vi "GPStest.vi"() -> ()   [LabVIEW 2019]
uses:
  <vilib>/LabVIEW Open Source Project/Data Manipulation/Scalar/FinalStringFormatting.vi
  <vilib>/Instr/_visa.llb/VISA Configure Serial Port (Instr).vi
  <vilib>/LabVIEW Open Source Project/Data Manipulation/Scalar/Get Decimal Separator.vi
  <vilib>/Utility/file.llb/Write Delimited Spreadsheet (string).vi
  <vilib>/LabVIEW Open Source Project/Data Manipulation/Scalar/OpenScalar.lvlib
panel:
  out "GPGSV":string
  out "number of message":string
  out "msg1":string
  out "Satelite in view":string
  in  "Satelite_id/elevation/azimuth/SNR 17":enum32{"Msg 1", "Msg 2", "Msg 3", "Msg 4"}(tab)
  out "Satelite_id/elevation/azimuth/SNR":string[](array[string])
  out "Satelite_id/elevation/azimuth/SNR 2":string[](array[string])
  out "Satelite_id/elevation/azimuth/SNR 3":string[](array[string])
  out "Satelite_id/elevation/azimuth/SNR 4":string[](array[string])
  out "Signal ID / Check sum":string[](array[string])
  out "Signal ID / Check sum 2":string[](array[string])
  out "Satelite_id/elevation/azimuth/SNR 8":string[](array[string])
  out "Satelite_id/elevation/azimuth/SNR 7":string[](array[string])
  out "Satelite_id/elevation/azimuth/SNR 6":string[](array[string])
  out "Satelite_id/elevation/azimuth/SNR 5":string[](array[string])
  out "Signal ID / Check sum 3":string[](array[string])
  out "Satelite_id/elevation/azimuth/SNR 12":string[](array[string])
  out "Satelite_id/elevation/azimuth/SNR 11":string[](array[string])
  out "Satelite_id/elevation/azimuth/SNR 10":string[](array[string])
  out "Satelite_id/elevation/azimuth/SNR 9":string[](array[string])
  out "Signal ID / Check sum 4":string[](array[string])
  out "Satelite_id/elevation/azimuth/SNR 16":string[](array[string])
  out "Satelite_id/elevation/azimuth/SNR 15":string[](array[string])
  out "Satelite_id/elevation/azimuth/SNR 14":string[](array[string])
  out "Satelite_id/elevation/azimuth/SNR 13":string[](array[string])
  out "GSA":string
  out "Operation Mode":string
  out "Navigation mode":string
  out "satelite used channel 1":string
  out "satelite used channel 2":string
  out "satelite used channel 3":string
  out "satelite used channel 4":string
  out "satelite used channel 5":string
  out "satelite used channel 6":string
  out "satelite used channel 7":string
  out "satelite used channel 8":string
  out "satelite used channel 9":string
  out "satelite used channel 10":string
  out "satelite used channel 11":string
  out "satelite used channel 12":string
  out "pdop":string
  out "hdop 2":string
  out "vdop":string
  out "System ID":string
  out "Checksum 3":string
  out "GGA 3":string
  out "UTC time":string
  out "Lat 3":string
  out "NS 2":string
  out "Long 2":string
  out "EW 2":string
  out "Pos_indicator":string
  out "Number of Satelite_used":string
  out "hdop":string
  out "msl_altitude":string
  out "altitude_units":string
  out "geoidal_Seperation":string
  out "Separation unit":string
  out "age of Diff corr":string
  out "diffStating":string
  out "Checksum 2":string
  out "VTG":string
  out "Course over Ground":string
  out "Reference":string
  out "Course over Ground (Magnetic)":string
  out "Reference2":string
  out "Speedover Ground (knots)":string
  out "Units1":string
  out "Speed over ground kph":string
  out "Units 2":string
  out "Position Mode 2":string
  out "Check sum 2":string
  out "Lat 2":string
  out "NS":string
  out "GLL":string
  out "Long 3":string
  out "EW":string
  out "Time":string
  out "Status 2":string
  out "Positioning mod":string
  out "Check sum":string
  out "Carriage return 2":string
  out "GBGSV 4":string
  out "number of message 4":string
  out "msg1 4":string
  out "Satelite in view 4":string
  in  "Satelite_id/elevation/azimuth/SNR 68":enum32{"Msg 1", "Msg 2", "Msg 3", "Msg 4"}(tab)
  out "Satelite_id/elevation/azimuth/SNR 55":string[](array[string])
  out "Satelite_id/elevation/azimuth/SNR 54":string[](array[string])
  out "Satelite_id/elevation/azimuth/SNR 53":string[](array[string])
  out "Satelite_id/elevation/azimuth/SNR 52":string[](array[string])
  out "Signal ID / Check sum 13":string[](array[string])
  out "Signal ID / Check sum 14":string[](array[string])
  out "Satelite_id/elevation/azimuth/SNR 59":string[](array[string])
  out "Satelite_id/elevation/azimuth/SNR 56":string[](array[string])
  out "Satelite_id/elevation/azimuth/SNR 57":string[](array[string])
  out "Satelite_id/elevation/azimuth/SNR 58":string[](array[string])
  out "Signal ID / Check sum 15":string[](array[string])
  out "Satelite_id/elevation/azimuth/SNR 63":string[](array[string])
  out "Satelite_id/elevation/azimuth/SNR 60":string[](array[string])
  out "Satelite_id/elevation/azimuth/SNR 61":string[](array[string])
  out "Satelite_id/elevation/azimuth/SNR 62":string[](array[string])
  out "Signal ID / Check sum 16":string[](array[string])
  out "Satelite_id/elevation/azimuth/SNR 67":string[](array[string])
  out "Satelite_id/elevation/azimuth/SNR 64":string[](array[string])
  out "Satelite_id/elevation/azimuth/SNR 65":string[](array[string])
  out "Satelite_id/elevation/azimuth/SNR 66":string[](array[string])
  out "GAGSV 3":string
  out "number of message 3":string
  out "msg1 3":string
  out "Satelite in view 3":string
  in  "Satelite_id/elevation/azimuth/SNR 51":enum32{"Msg 1", "Msg 2", "Msg 3", "Msg 4"}(tab)
  out "Satelite_id/elevation/azimuth/SNR 38":string[](array[string])
  out "Satelite_id/elevation/azimuth/SNR 37":string[](array[string])
  out "Satelite_id/elevation/azimuth/SNR 36":string[](array[string])
  out "Satelite_id/elevation/azimuth/SNR 35":string[](array[string])
  out "Signal ID / Check sum 9":string[](array[string])
  out "Signal ID / Check sum 10":string[](array[string])
  out "Satelite_id/elevation/azimuth/SNR 42":string[](array[string])
  out "Satelite_id/elevation/azimuth/SNR 39":string[](array[string])
  out "Satelite_id/elevation/azimuth/SNR 40":string[](array[string])
  out "Satelite_id/elevation/azimuth/SNR 41":string[](array[string])
  out "Signal ID / Check sum 11":string[](array[string])
  out "Satelite_id/elevation/azimuth/SNR 46":string[](array[string])
  out "Satelite_id/elevation/azimuth/SNR 43":string[](array[string])
  out "Satelite_id/elevation/azimuth/SNR 44":string[](array[string])
  out "Satelite_id/elevation/azimuth/SNR 45":string[](array[string])
  out "Signal ID / Check sum 12":string[](array[string])
  out "Satelite_id/elevation/azimuth/SNR 50":string[](array[string])
  out "Satelite_id/elevation/azimuth/SNR 47":string[](array[string])
  out "Satelite_id/elevation/azimuth/SNR 48":string[](array[string])
  out "Satelite_id/elevation/azimuth/SNR 49":string[](array[string])
  out "GLGSV 2":string
  out "number of message 2":string
  out "msg1 2":string
  out "Satelite in view 2":string
  in  "Satelite_id/elevation/azimuth/SNR 34":enum32{"Msg 1", "Msg 2", "Msg 3", "Msg 4"}(tab)
  out "Satelite_id/elevation/azimuth/SNR 21":string[](array[string])
  out "Satelite_id/elevation/azimuth/SNR 20":string[](array[string])
  out "Satelite_id/elevation/azimuth/SNR 19":string[](array[string])
  out "Satelite_id/elevation/azimuth/SNR 18":string[](array[string])
  out "Signal ID / Check sum 5":string[](array[string])
  out "Signal ID / Check sum 6":string[](array[string])
  out "Satelite_id/elevation/azimuth/SNR 25":string[](array[string])
  out "Satelite_id/elevation/azimuth/SNR 22":string[](array[string])
  out "Satelite_id/elevation/azimuth/SNR 23":string[](array[string])
  out "Satelite_id/elevation/azimuth/SNR 24":string[](array[string])
  out "Signal ID / Check sum 7":string[](array[string])
  out "Satelite_id/elevation/azimuth/SNR 29":string[](array[string])
  out "Satelite_id/elevation/azimuth/SNR 26":string[](array[string])
  out "Satelite_id/elevation/azimuth/SNR 27":string[](array[string])
  out "Satelite_id/elevation/azimuth/SNR 28":string[](array[string])
  out "Signal ID / Check sum 8":string[](array[string])
  out "Satelite_id/elevation/azimuth/SNR 33":string[](array[string])
  out "Satelite_id/elevation/azimuth/SNR 30":string[](array[string])
  out "Satelite_id/elevation/azimuth/SNR 31":string[](array[string])
  out "Satelite_id/elevation/azimuth/SNR 32":string[](array[string])
  out "UTC Time":string
  out "Status":string
  out "Lat":string
  out "N/S":string
  out "Long":string
  out "E/W":string
  out "Speed over ground[knot]":string
  out "Course over Ground [Degrees]":string
  out "date[ddmmyy]":string
  out "Mode":string
  out "xxRMC":string
  out "NavStatus":string
  out "Checksum":string
  out "Carriage return":string
  in  "stop":bool
  in  "error in (no error) 2":errorcluster
  out "read buffer":string
  out "Array":string[](array[string])
  out "VISA Refnum":refnum<visa-resource-name>
  out "error out":errorcluster
  out "Raw output from GPS":string
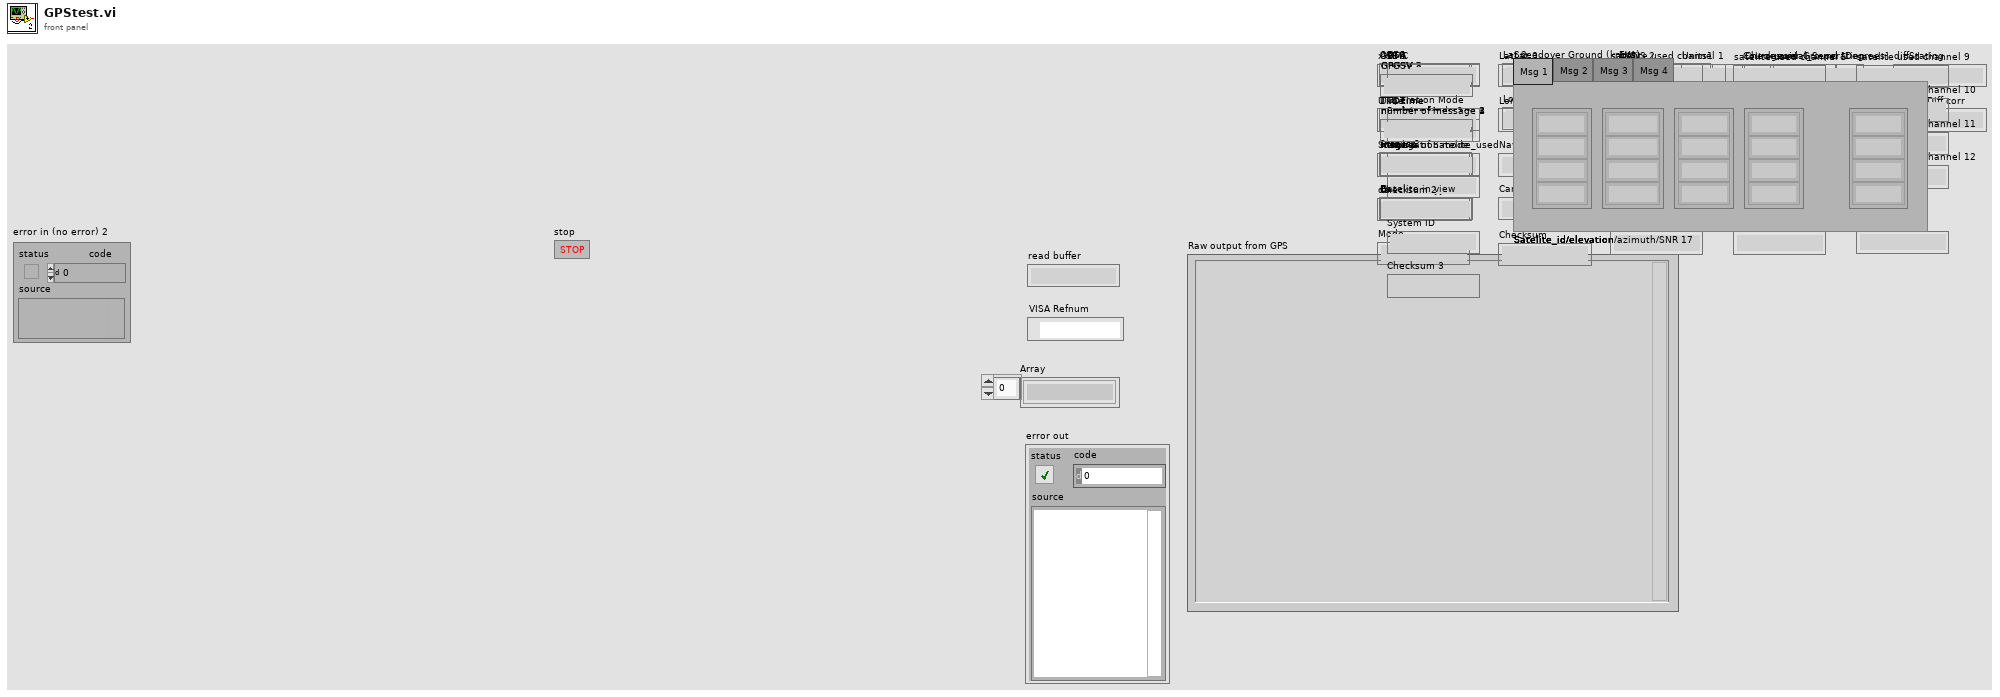
[diagram p1: front panel]
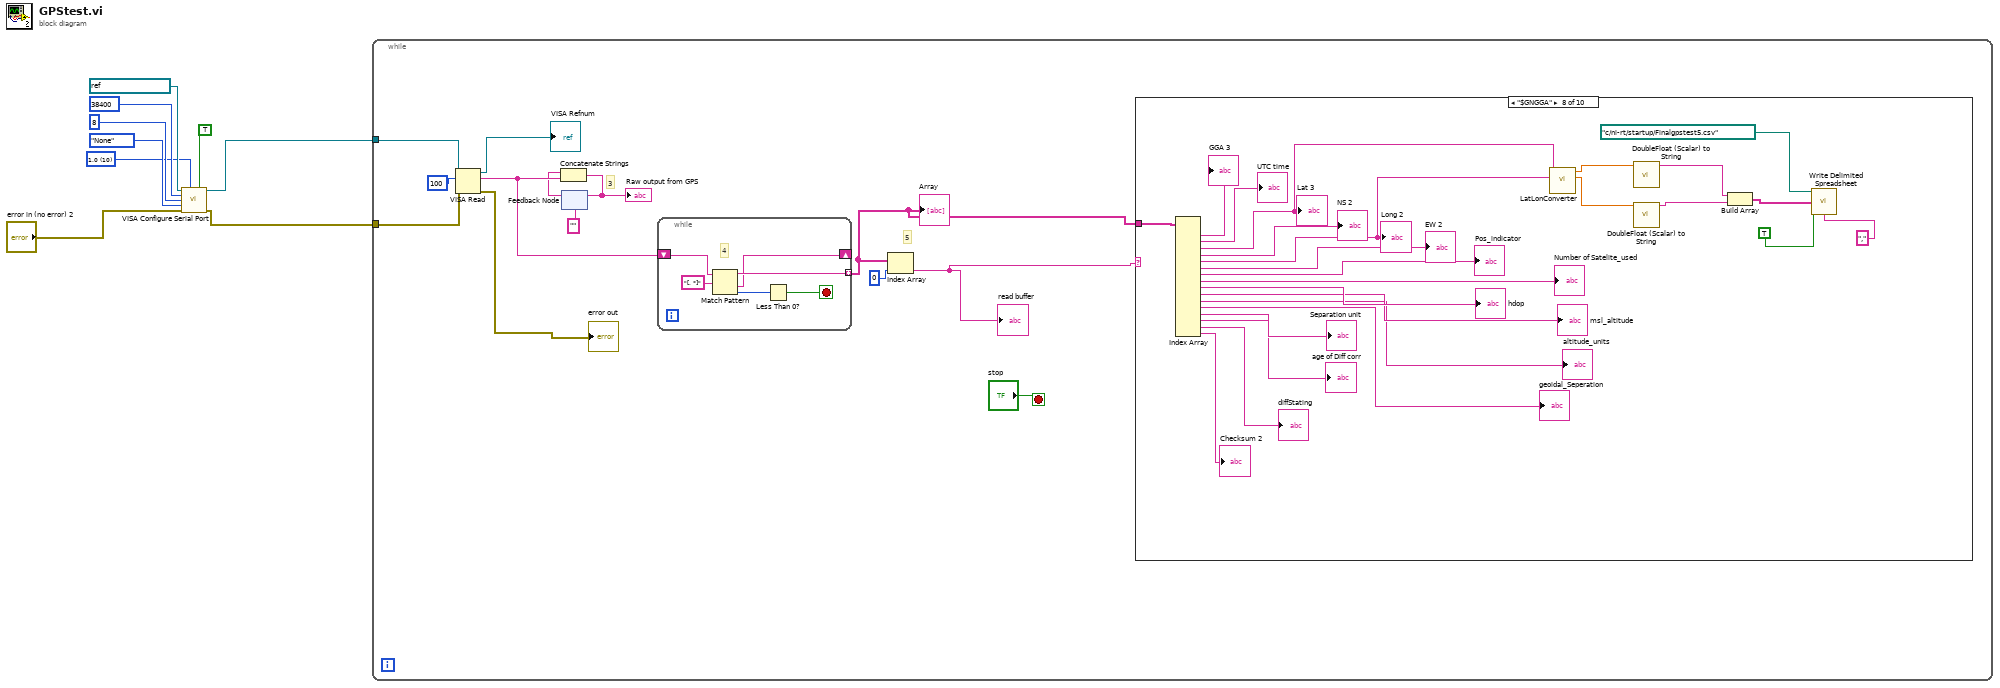
[diagram p0: block diagram]
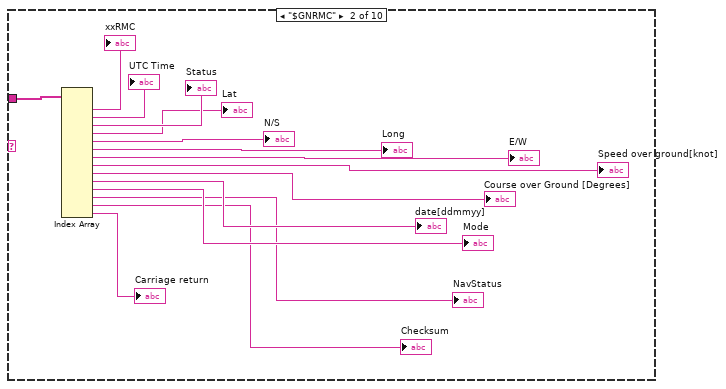
[diagram p3: hidden frame]
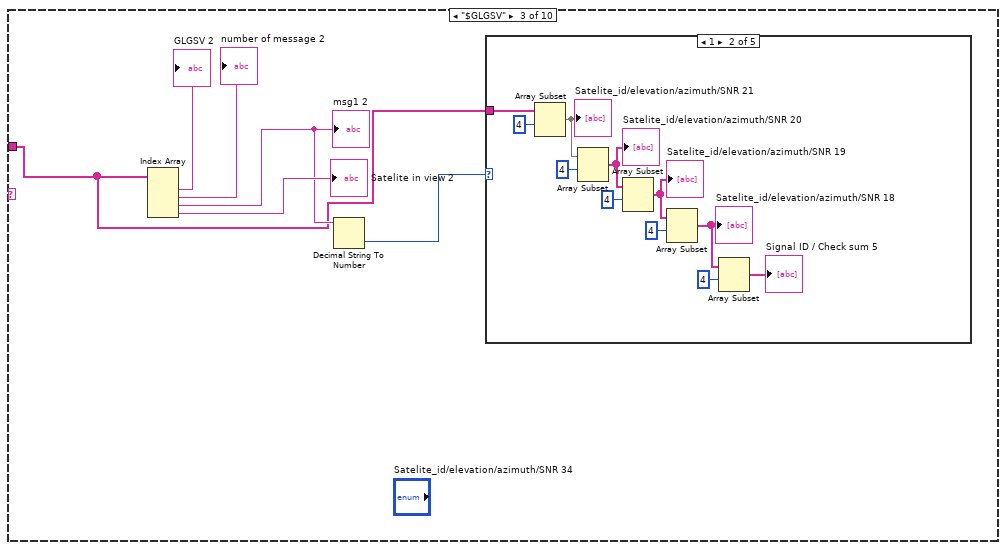
[diagram p4: hidden frame]
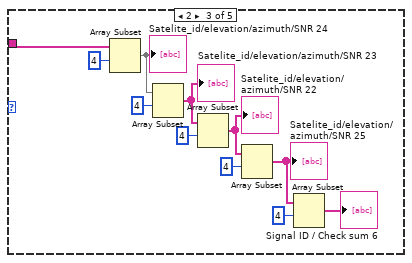
[diagram p6: hidden frame]
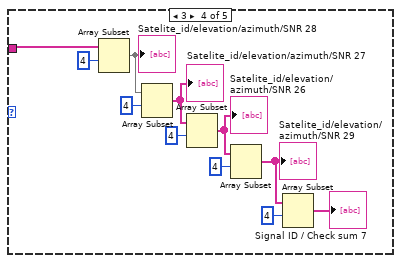
[diagram p7: hidden frame]
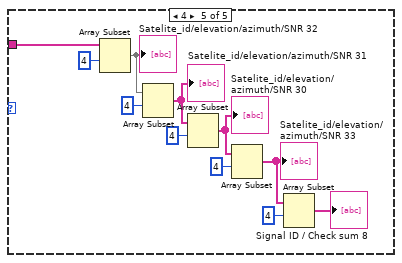
[diagram p8: hidden frame]
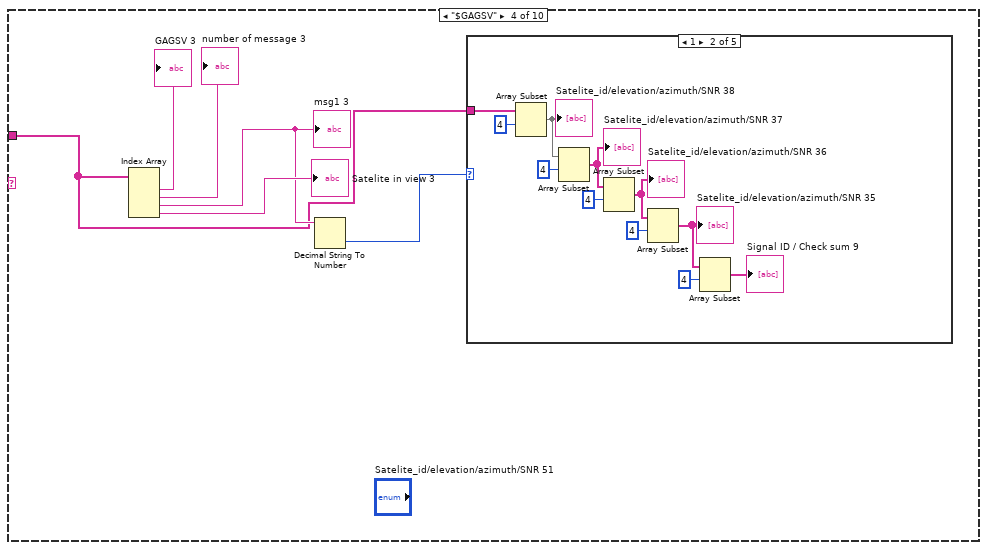
[diagram p9: hidden frame]
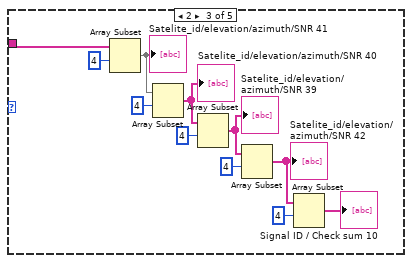
[diagram p11: hidden frame]
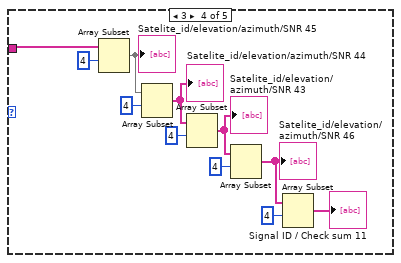
[diagram p12: hidden frame]
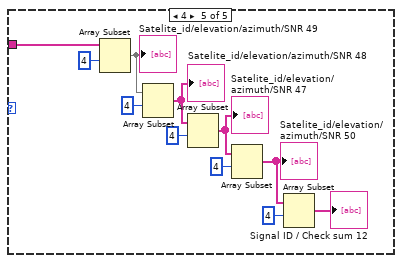
[diagram p13: hidden frame]
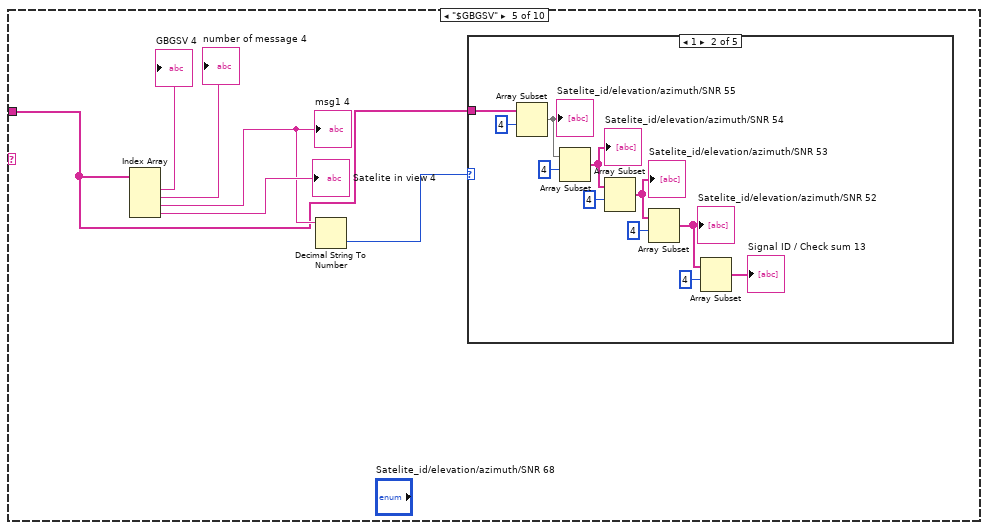
[diagram p14: hidden frame]
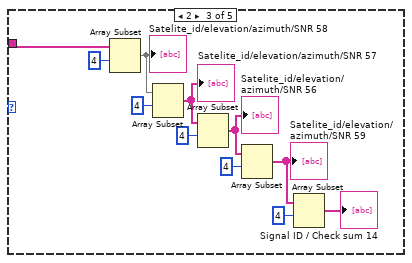
[diagram p16: hidden frame]
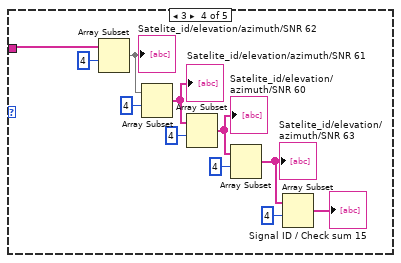
[diagram p17: hidden frame]
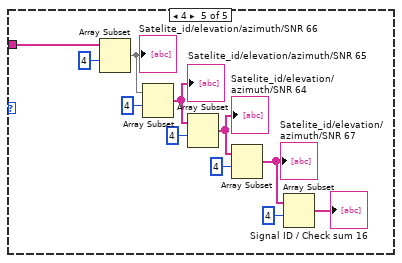
[diagram p18: hidden frame]
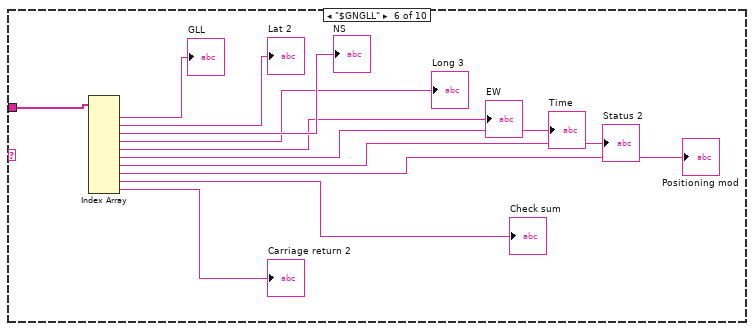
[diagram p19: hidden frame]
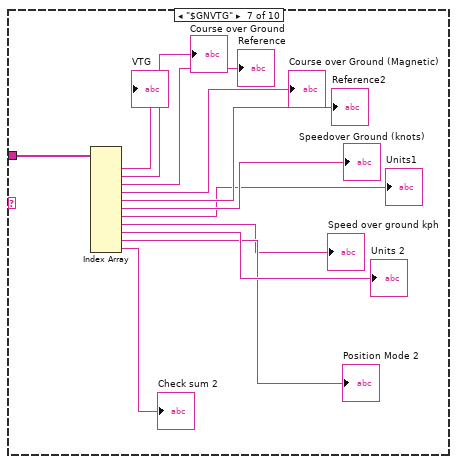
[diagram p20: hidden frame]
diagram:
  w4 = u16 10 items=["1.0"=10, "1.5"=15, "2.0"=20] ("stop bits (10: 1 bit)")
  n1 = call-poly "VISA Configure Serial Port"("VISA resource name"=refnum<visa-resource-name> "ASRL1::INSTR", "Enable Termination\nChar (T)"=TRUE ("Enable Termination\nChar (T)"), "baud rate (9600)"=u32 38400, "data bits (8)"=u16 8, "parity (0:none)"=enum16{"None", "Odd", "Even", "Mark", "Space"}."None", "error in (no error)"="error in (no error) 2", "stop bits (10: 1 bit)"=w4) -> ("VISA resource name out"=w3:refnum<visa-resource-name>, "error out"=w1:errorcluster)  [unwired: 7 in]
  n2 = while {
    tunnel: w3 -> [w15]
    tunnel: w1 -> [w14]
    stop <- "stop" stop-if-true
    # "5"
    # "3"
    n3 = VISA Read(VISA resource name=w15, byte count=u32 100, error in (no error)=w14) -> (VISA resource name out=→"VISA Refnum":refnum<visa-resource-name>, read buffer=w20:string, error out=→"error out":errorcluster)  [unwired: 1 out]
    n4 = feedback #1("") -> (w18:string)
    n5 = Concatenate Strings(w18, w20) -> (w17:string)
    "Raw output from GPS" <- w17
    n6 = feedback-in #1(w17) -> ()
    n7 = while {
      tunnel: [w310] -> w11 mode=indexing
      shift-right: [w309] -> _
      shift-left: w20 -> [w312]
      stop <- w307 stop-if-true
      # "4"
      n8 = Match Pattern(string=w312, regular expression="[, *]") -> (before substring=w310:string, after substring=w309:string, offset past match=w308:i32)  [unwired: 1 in, 1 out]
      n9 = Less Than 0?(x=w308) -> (x < 0?=w307:bool)
    }
    "Array" <- w11
    n10 = Index Array(array=w11, index=0) -> (element=w10:string)
    "read buffer" <- w10
    n11 = case shown="\"$GNGGA\"" w10 {
      tunnel: w11 -> [_ w37 w38 w88 w138 w198 w210 w235 w256 w257]
      frame "False", Default {
      }
      frame "$GNRMC" {
        n12 = Index Array(array=w37) -> (element #1=→"xxRMC":string, element #2=→"UTC Time":string, element #3=→"Status":string, element #4=→"Lat":string, element #5=→"N/S":string, element #6=→"Long":string, element #7=→"E/W":string, element #8=→"Speed over ground[knot]":string, element #9=→"Course over Ground [Degrees]":string, element #10=→"date[ddmmyy]":string, element #11=→"Mode":string, element #12=→"NavStatus":string, element #13=→"Checksum":string, element #14=→"Carriage return":string)  [unwired: 14 in]
      }
      frame "$GLGSV" {
        n13 = Index Array(array=w38) -> (element #1=→"GLGSV 2":string, element #2=→"number of message 2":string, element #3=w40:string, element #4=→"Satelite in view 2":string)  [unwired: 4 in]
        "msg1 2" <- w40
        n14 = Decimal String To Number(string=w40) -> (number=w39:i32)  [unwired: 2 in, 1 out]
        n15 = case shown="1" w39 {
          tunnel: w38 -> [_ w45 w55 w66 w77]
          frame 0, Default {
          }
          frame 1 {
            n16 = Array Subset(array=w45, index=4) -> (w50:string[])  [unwired: 1 in]
            "Satelite_id/elevation/azimuth/SNR 21" <- w50
            n17 = Array Subset(array=w50, index=4) -> (w51:string[])  [unwired: 1 in]
            "Satelite_id/elevation/azimuth/SNR 20" <- w51
            n18 = Array Subset(array=w51, index=4) -> (w52:string[])  [unwired: 1 in]
            "Satelite_id/elevation/azimuth/SNR 19" <- w52
            n19 = Array Subset(array=w52, index=4) -> (w54:string[])  [unwired: 1 in]
            "Satelite_id/elevation/azimuth/SNR 18" <- w54
            n20 = Array Subset(array=w54, index=4) -> (→"Signal ID / Check sum 5":string[])  [unwired: 1 in]
          }
          frame 2 {
            n21 = Array Subset(array=w55, index=4) -> (w61:string[])  [unwired: 1 in]
            "Satelite_id/elevation/azimuth/SNR 24" <- w61
            n22 = Array Subset(array=w61, index=4) -> (w62:string[])  [unwired: 1 in]
            "Satelite_id/elevation/azimuth/SNR 23" <- w62
            n23 = Array Subset(array=w62, index=4) -> (w63:string[])  [unwired: 1 in]
            "Satelite_id/elevation/azimuth/SNR 22" <- w63
            n24 = Array Subset(array=w63, index=4) -> (w65:string[])  [unwired: 1 in]
            "Satelite_id/elevation/azimuth/SNR 25" <- w65
            n25 = Array Subset(array=w65, index=4) -> (→"Signal ID / Check sum 6":string[])  [unwired: 1 in]
          }
          frame 3 {
            n26 = Array Subset(array=w66, index=4) -> (w72:string[])  [unwired: 1 in]
            "Satelite_id/elevation/azimuth/SNR 28" <- w72
            n27 = Array Subset(array=w72, index=4) -> (w73:string[])  [unwired: 1 in]
            "Satelite_id/elevation/azimuth/SNR 27" <- w73
            n28 = Array Subset(array=w73, index=4) -> (w74:string[])  [unwired: 1 in]
            "Satelite_id/elevation/azimuth/SNR 26" <- w74
            n29 = Array Subset(array=w74, index=4) -> (w76:string[])  [unwired: 1 in]
            "Satelite_id/elevation/azimuth/SNR 29" <- w76
            n30 = Array Subset(array=w76, index=4) -> (→"Signal ID / Check sum 7":string[])  [unwired: 1 in]
          }
          frame 4 {
            n31 = Array Subset(array=w77, index=4) -> (w83:string[])  [unwired: 1 in]
            "Satelite_id/elevation/azimuth/SNR 32" <- w83
            n32 = Array Subset(array=w83, index=4) -> (w84:string[])  [unwired: 1 in]
            "Satelite_id/elevation/azimuth/SNR 31" <- w84
            n33 = Array Subset(array=w84, index=4) -> (w85:string[])  [unwired: 1 in]
            "Satelite_id/elevation/azimuth/SNR 30" <- w85
            n34 = Array Subset(array=w85, index=4) -> (w87:string[])  [unwired: 1 in]
            "Satelite_id/elevation/azimuth/SNR 33" <- w87
            n35 = Array Subset(array=w87, index=4) -> (→"Signal ID / Check sum 8":string[])  [unwired: 1 in]
          }
        }
      }
      frame "$GAGSV" {
        n36 = Index Array(array=w88) -> (element #1=→"GAGSV 3":string, element #2=→"number of message 3":string, element #3=w90:string, element #4=→"Satelite in view 3":string)  [unwired: 4 in]
        "msg1 3" <- w90
        n37 = Decimal String To Number(string=w90) -> (number=w89:i32)  [unwired: 2 in, 1 out]
        n38 = case shown="1" w89 {
          tunnel: w88 -> [_ w95 w105 w116 w127]
          frame 0, Default {
          }
          frame 1 {
            n39 = Array Subset(array=w95, index=4) -> (w100:string[])  [unwired: 1 in]
            "Satelite_id/elevation/azimuth/SNR 38" <- w100
            n40 = Array Subset(array=w100, index=4) -> (w101:string[])  [unwired: 1 in]
            "Satelite_id/elevation/azimuth/SNR 37" <- w101
            n41 = Array Subset(array=w101, index=4) -> (w102:string[])  [unwired: 1 in]
            "Satelite_id/elevation/azimuth/SNR 36" <- w102
            n42 = Array Subset(array=w102, index=4) -> (w104:string[])  [unwired: 1 in]
            "Satelite_id/elevation/azimuth/SNR 35" <- w104
            n43 = Array Subset(array=w104, index=4) -> (→"Signal ID / Check sum 9":string[])  [unwired: 1 in]
          }
          frame 2 {
            n44 = Array Subset(array=w105, index=4) -> (w111:string[])  [unwired: 1 in]
            "Satelite_id/elevation/azimuth/SNR 41" <- w111
            n45 = Array Subset(array=w111, index=4) -> (w112:string[])  [unwired: 1 in]
            "Satelite_id/elevation/azimuth/SNR 40" <- w112
            n46 = Array Subset(array=w112, index=4) -> (w113:string[])  [unwired: 1 in]
            "Satelite_id/elevation/azimuth/SNR 39" <- w113
            n47 = Array Subset(array=w113, index=4) -> (w115:string[])  [unwired: 1 in]
            "Satelite_id/elevation/azimuth/SNR 42" <- w115
            n48 = Array Subset(array=w115, index=4) -> (→"Signal ID / Check sum 10":string[])  [unwired: 1 in]
          }
          frame 3 {
            n49 = Array Subset(array=w116, index=4) -> (w122:string[])  [unwired: 1 in]
            "Satelite_id/elevation/azimuth/SNR 45" <- w122
            n50 = Array Subset(array=w122, index=4) -> (w123:string[])  [unwired: 1 in]
            "Satelite_id/elevation/azimuth/SNR 44" <- w123
            n51 = Array Subset(array=w123, index=4) -> (w124:string[])  [unwired: 1 in]
            "Satelite_id/elevation/azimuth/SNR 43" <- w124
            n52 = Array Subset(array=w124, index=4) -> (w126:string[])  [unwired: 1 in]
            "Satelite_id/elevation/azimuth/SNR 46" <- w126
            n53 = Array Subset(array=w126, index=4) -> (→"Signal ID / Check sum 11":string[])  [unwired: 1 in]
          }
          frame 4 {
            n54 = Array Subset(array=w127, index=4) -> (w133:string[])  [unwired: 1 in]
            "Satelite_id/elevation/azimuth/SNR 49" <- w133
            n55 = Array Subset(array=w133, index=4) -> (w134:string[])  [unwired: 1 in]
            "Satelite_id/elevation/azimuth/SNR 48" <- w134
            n56 = Array Subset(array=w134, index=4) -> (w135:string[])  [unwired: 1 in]
            "Satelite_id/elevation/azimuth/SNR 47" <- w135
            n57 = Array Subset(array=w135, index=4) -> (w137:string[])  [unwired: 1 in]
            "Satelite_id/elevation/azimuth/SNR 50" <- w137
            n58 = Array Subset(array=w137, index=4) -> (→"Signal ID / Check sum 12":string[])  [unwired: 1 in]
          }
        }
      }
      frame "$GBGSV" {
        n59 = Index Array(array=w138) -> (element #1=→"GBGSV 4":string, element #2=→"number of message 4":string, element #3=w140:string, element #4=→"Satelite in view 4":string)  [unwired: 4 in]
        "msg1 4" <- w140
        n60 = Decimal String To Number(string=w140) -> (number=w139:i32)  [unwired: 2 in, 1 out]
        n61 = case shown="1" w139 {
          tunnel: w138 -> [_ w145 w155 w166 w177]
          frame 0, Default {
          }
          frame 1 {
            n62 = Array Subset(array=w145, index=4) -> (w150:string[])  [unwired: 1 in]
            "Satelite_id/elevation/azimuth/SNR 55" <- w150
            n63 = Array Subset(array=w150, index=4) -> (w151:string[])  [unwired: 1 in]
            "Satelite_id/elevation/azimuth/SNR 54" <- w151
            n64 = Array Subset(array=w151, index=4) -> (w152:string[])  [unwired: 1 in]
            "Satelite_id/elevation/azimuth/SNR 53" <- w152
            n65 = Array Subset(array=w152, index=4) -> (w154:string[])  [unwired: 1 in]
            "Satelite_id/elevation/azimuth/SNR 52" <- w154
            n66 = Array Subset(array=w154, index=4) -> (→"Signal ID / Check sum 13":string[])  [unwired: 1 in]
          }
          frame 2 {
            n67 = Array Subset(array=w155, index=4) -> (w161:string[])  [unwired: 1 in]
            "Satelite_id/elevation/azimuth/SNR 58" <- w161
            n68 = Array Subset(array=w161, index=4) -> (w162:string[])  [unwired: 1 in]
            "Satelite_id/elevation/azimuth/SNR 57" <- w162
            n69 = Array Subset(array=w162, index=4) -> (w163:string[])  [unwired: 1 in]
            "Satelite_id/elevation/azimuth/SNR 56" <- w163
            n70 = Array Subset(array=w163, index=4) -> (w165:string[])  [unwired: 1 in]
            "Satelite_id/elevation/azimuth/SNR 59" <- w165
            n71 = Array Subset(array=w165, index=4) -> (→"Signal ID / Check sum 14":string[])  [unwired: 1 in]
          }
          frame 3 {
            n72 = Array Subset(array=w166, index=4) -> (w172:string[])  [unwired: 1 in]
            "Satelite_id/elevation/azimuth/SNR 62" <- w172
            n73 = Array Subset(array=w172, index=4) -> (w173:string[])  [unwired: 1 in]
            "Satelite_id/elevation/azimuth/SNR 61" <- w173
            n74 = Array Subset(array=w173, index=4) -> (w174:string[])  [unwired: 1 in]
            "Satelite_id/elevation/azimuth/SNR 60" <- w174
            n75 = Array Subset(array=w174, index=4) -> (w176:string[])  [unwired: 1 in]
            "Satelite_id/elevation/azimuth/SNR 63" <- w176
            n76 = Array Subset(array=w176, index=4) -> (→"Signal ID / Check sum 15":string[])  [unwired: 1 in]
          }
          frame 4 {
            n77 = Array Subset(array=w177, index=4) -> (w183:string[])  [unwired: 1 in]
            "Satelite_id/elevation/azimuth/SNR 66" <- w183
            n78 = Array Subset(array=w183, index=4) -> (w184:string[])  [unwired: 1 in]
            "Satelite_id/elevation/azimuth/SNR 65" <- w184
            n79 = Array Subset(array=w184, index=4) -> (w185:string[])  [unwired: 1 in]
            "Satelite_id/elevation/azimuth/SNR 64" <- w185
            n80 = Array Subset(array=w185, index=4) -> (w187:string[])  [unwired: 1 in]
            "Satelite_id/elevation/azimuth/SNR 67" <- w187
            n81 = Array Subset(array=w187, index=4) -> (→"Signal ID / Check sum 16":string[])  [unwired: 1 in]
          }
        }
      }
      frame "$GNGLL" {
        n82 = Index Array(array=w198) -> (element #1=→"GLL":string, element #2=→"Lat 2":string, element #3=→"NS":string, element #4=→"Long 3":string, element #5=→"EW":string, element #6=→"Time":string, element #7=→"Status 2":string, element #8=→"Positioning mod":string, element #9=→"Check sum":string, element #10=→"Carriage return 2":string)  [unwired: 10 in]
      }
      frame "$GNVTG" {
        n83 = Index Array(array=w210) -> (element #1=→"VTG":string, element #2=→"Course over Ground":string, element #3=→"Reference":string, element #4=→"Course over Ground (Magnetic)":string, element #5=→"Reference2":string, element #6=→"Speedover Ground (knots)":string, element #7=→"Units1":string, element #8=→"Speed over ground kph":string, element #9=→"Units 2":string, element #10=→"Position Mode 2":string, element #11=→"Check sum 2":string)  [unwired: 11 in]
      }
      frame "$GNGGA" {
        n84 = Index Array(array=w235) -> (element #1=→"GGA 3":string, element #2=→"UTC time":string, element #3=w217:string, element #4=→"NS 2":string, element #5=w216:string, element #6=→"EW 2":string, element #7=→"Pos_indicator":string, element #8=→"Number of Satelite_used":string, element #9=→"hdop":string, element #10=→"msl_altitude":string, element #11=→"altitude_units":string, element #12=→"geoidal_Seperation":string, element #13=→"Separation unit":string, element #14=→"age of Diff corr":string, element #15=→"diffStating":string, element #16=→"Checksum 2":string)  [unwired: 16 in]
        "Lat 3" <- w217
        "Long 2" <- w216
        n85 = call "LatLonConverter.vi"("lon (GPS string)"=w216, "lat (GPS string)"=w217) -> ("lon (degrees)"=w214:dbl, "lat (degrees)"=w215:dbl)  [unwired: 8 in]
        n86 = call <vilib>:"DoubleFloat (Scalar) to String.vi"("Value (Double)"=w215) -> ("Value (String)"=w212:string)  [unwired: 10 in]
        n87 = call <vilib>:"DoubleFloat (Scalar) to String.vi"("Value (Double)"=w214) -> ("Value (String)"=w213:string)  [unwired: 10 in]
        n88 = Build Array(w212, w213) -> (w211:string[])
        n89 = call-poly <vilib>:"Write Delimited Spreadsheet.vi"("file path (dialog if empty)"=path "c:/ni-rt/startup/Finalgpstest5.csv", "1D data"=w211, "append to file? (new file:F)"=TRUE, "delimiter (\\t)"="," ("delimiter (\\t)")) -> ()  [unwired: 10 in, 2 out]
      }
      frame "$GNGSA" {
        n90 = Index Array(array=w256) -> (element #1=→"GSA":string, element #2=→"Operation Mode":string, element #3=→"Navigation mode":string, element #4=→"satelite used channel 1":string, element #5=→"satelite used channel 2":string, element #6=→"satelite used channel 3":string, element #7=→"satelite used channel 4":string, element #8=→"satelite used channel 5":string, element #9=→"satelite used channel 6":string, element #10=→"satelite used channel 7":string, element #11=→"satelite used channel 8":string, element #12=→"satelite used channel 9":string, element #13=→"satelite used channel 10":string, element #14=→"satelite used channel 11":string, element #15=→"satelite used channel 12":string, element #16=→"pdop":string, element #17=→"hdop 2":string, element #18=→"vdop":string, element #19=→"System ID":string, element #20=→"Checksum 3":string)  [unwired: 20 in]
      }
      frame "$GPGSV" {
        n91 = Index Array(array=w257) -> (element #1=→"GPGSV":string, element #2=→"number of message":string, element #3=w259:string, element #4=→"Satelite in view":string)  [unwired: 4 in]
        "msg1" <- w259
        n92 = Decimal String To Number(string=w259) -> (number=w258:i32)  [unwired: 2 in, 1 out]
        n93 = case shown="1" w258 {
          tunnel: w257 -> [_ w264 w274 w285 w296]
          frame 0, Default {
          }
          frame 1 {
            n94 = Array Subset(array=w264, index=4) -> (w269:string[])  [unwired: 1 in]
            "Satelite_id/elevation/azimuth/SNR" <- w269
            n95 = Array Subset(array=w269, index=4) -> (w270:string[])  [unwired: 1 in]
            "Satelite_id/elevation/azimuth/SNR 2" <- w270
            n96 = Array Subset(array=w270, index=4) -> (w271:string[])  [unwired: 1 in]
            "Satelite_id/elevation/azimuth/SNR 3" <- w271
            n97 = Array Subset(array=w271, index=4) -> (w273:string[])  [unwired: 1 in]
            "Satelite_id/elevation/azimuth/SNR 4" <- w273
            n98 = Array Subset(array=w273, index=4) -> (→"Signal ID / Check sum":string[])  [unwired: 1 in]
          }
          frame 2 {
            n99 = Array Subset(array=w274, index=4) -> (w280:string[])  [unwired: 1 in]
            "Satelite_id/elevation/azimuth/SNR 5" <- w280
            n100 = Array Subset(array=w280, index=4) -> (w281:string[])  [unwired: 1 in]
            "Satelite_id/elevation/azimuth/SNR 6" <- w281
            n101 = Array Subset(array=w281, index=4) -> (w282:string[])  [unwired: 1 in]
            "Satelite_id/elevation/azimuth/SNR 7" <- w282
            n102 = Array Subset(array=w282, index=4) -> (w284:string[])  [unwired: 1 in]
            "Satelite_id/elevation/azimuth/SNR 8" <- w284
            n103 = Array Subset(array=w284, index=4) -> (→"Signal ID / Check sum 2":string[])  [unwired: 1 in]
          }
          frame 3 {
            n104 = Array Subset(array=w285, index=4) -> (w291:string[])  [unwired: 1 in]
            "Satelite_id/elevation/azimuth/SNR 9" <- w291
            n105 = Array Subset(array=w291, index=4) -> (w292:string[])  [unwired: 1 in]
            "Satelite_id/elevation/azimuth/SNR 10" <- w292
            n106 = Array Subset(array=w292, index=4) -> (w293:string[])  [unwired: 1 in]
            "Satelite_id/elevation/azimuth/SNR 11" <- w293
            n107 = Array Subset(array=w293, index=4) -> (w295:string[])  [unwired: 1 in]
            "Satelite_id/elevation/azimuth/SNR 12" <- w295
            n108 = Array Subset(array=w295, index=4) -> (→"Signal ID / Check sum 3":string[])  [unwired: 1 in]
          }
          frame 4 {
            n109 = Array Subset(array=w296, index=4) -> (w302:string[])  [unwired: 1 in]
            "Satelite_id/elevation/azimuth/SNR 13" <- w302
            n110 = Array Subset(array=w302, index=4) -> (w303:string[])  [unwired: 1 in]
            "Satelite_id/elevation/azimuth/SNR 14" <- w303
            n111 = Array Subset(array=w303, index=4) -> (w304:string[])  [unwired: 1 in]
            "Satelite_id/elevation/azimuth/SNR 15" <- w304
            n112 = Array Subset(array=w304, index=4) -> (w306:string[])  [unwired: 1 in]
            "Satelite_id/elevation/azimuth/SNR 16" <- w306
            n113 = Array Subset(array=w306, index=4) -> (→"Signal ID / Check sum 4":string[])  [unwired: 1 in]
          }
        }
      }
    }
  }
